vi "Coherent decode mode.vi"(11 "Mode string":string) -> (3 "Mode Desc.":string)   [LabVIEW 2017]
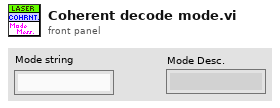
[diagram p1: front panel]
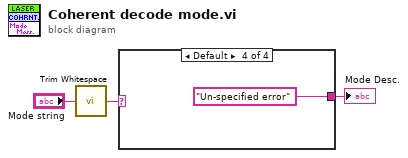
[diagram p0: block diagram]
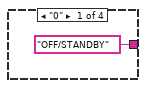
[diagram p2: hidden frame]
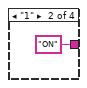
[diagram p3: hidden frame]
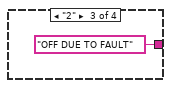
[diagram p4: hidden frame]
diagram:
  n1 = call <vilib>:"Trim Whitespace.vi"("string"="Mode string") -> ("trimmed string"=w2:string)  [unwired: 1 in]
  n2 = case shown="Default" w2 {
    tunnel: ["OFF/STANDBY" "ON" "OFF DUE TO FAULT" "Un-specified error"] -> w1
    frame "0" {
    }
    frame "1" {
    }
    frame "2" {
    }
    frame Default {
    }
  }
  "Mode Desc." <- w1
